vi "ini_Cylinder.vi"(8 "error IO":errorcluster) -> (0 "error out":errorcluster)   [LabVIEW 2017]
uses:
  Ctrls/AlarmIndex.ctl
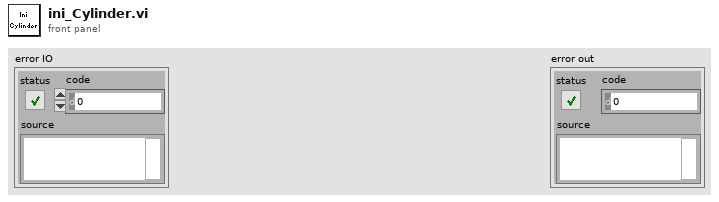
[diagram p1: front panel]
types:
  T1 = typedef "AlarmIndex.ctl" = enum16{"E-Stop", "Safety light grid", "UUT Sealing Cylinder HomePoint", "UUT Sealing Cylinder WorkPoint", "Orifice fixed Cylinder L HomePoint", "Orifice fixed Cylinder L WorkPoint", "Orifice fixed Cylinder R HomePoint", "Orifice fixed Cylinder R WorkPoint", "UUT Cylinder HomePoint", "UUT Cylinder WorkPoint", "Carrier fixed Cylinder L HomePoint", "Carrier fixed Cylinder L WorkPoint", "Carrier fixed Cylinder R HomePoint", "Carrier fixed Cylinder R WorkPoint", "Probe Cylinder HomePoint", "Probe Cylinder WorkPoint", "Motor Error", "Test Error"}
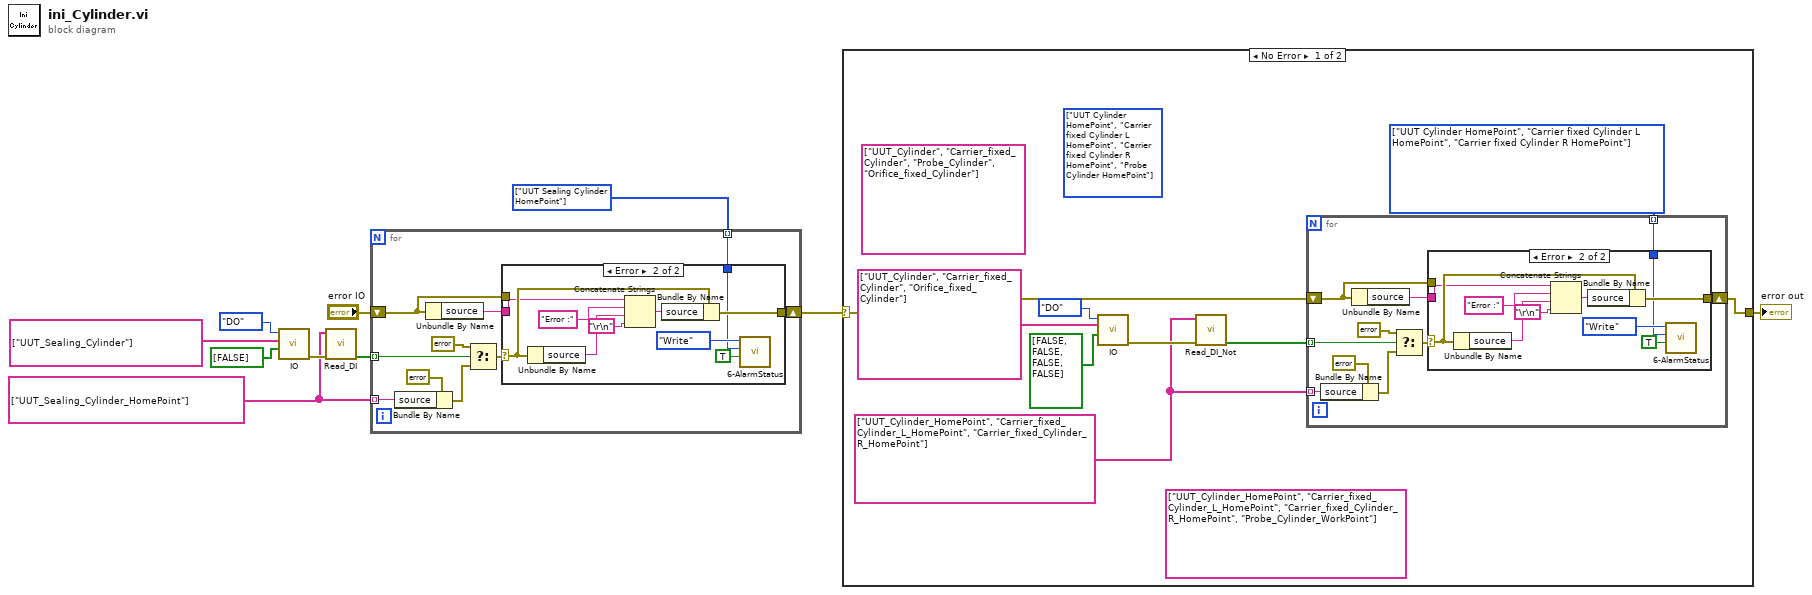
[diagram p0: block diagram]
diagram:
  w4 = T1[] [enum."UUT Sealing Cylinder HomePoint"] items=["E-Stop", "Safety light grid", "UUT Sealing Cylinder HomePoint", "UUT Sealing Cylinder WorkPoint", "Orifice fixed Cylinder L HomePoint", "Orifice fixed Cylinder L WorkPoint", "Orifice fixed Cylinder R HomePoint", "Orifice fixed Cylinder R WorkPoint", "UUT Cylinder HomePoint", "UUT Cylinder WorkPoint", "Carrier fixed Cylinder L HomePoint", "Carrier fixed Cylinder L WorkPoint", "Carrier fixed Cylinder R HomePoint", "Carrier fixed Cylinder R WorkPoint", "Probe Cylinder HomePoint", "Probe Cylinder WorkPoint", "Motor Error", "Test Error"]
  w5 = string[] ["UUT_Sealing_Cylinder_HomePoint"] ("IO Name")
  n1 = call "IO.vi"("DO DATA"=bool[] [FALSE] ("Writel_IO"), "IO Name"=string[] ["UUT_Sealing_Cylinder"], "IO?"=enum16{"DI", "DO"}."DO") -> ("error out"=w8:errorcluster)  [unwired: 7 in, 1 out]
  n2 = call "Read_DI.vi"("error in (no error)"=w8, "Name"=w5) -> ("DI"=w6:bool[])  [unwired: 8 in, 1 out]
  n3 = for {
    shift-right: [w16] -> w3
    shift-left: "error IO" -> [w12]
    tunnel: w6 -> [w18] mode=indexing
    tunnel: w5 -> [w15] mode=indexing
    tunnel: w4 -> [w11] mode=indexing
    n4 = Bundle By Name(cluster=errorcluster {"status"=TRUE, "code"=0, "source"=""} ("error out"), "source"=w15) -> (w17:errorcluster)
    n5 = Unbundle By Name(w12) -> ("source"=w13:string)
    n6 = Select(t=errorcluster {"status"=FALSE, "code"=0, "source"=""}, s=w18, f=w17) -> (s? t:f=w19:errorcluster)
    n7 = case shown="Error" w19 {
      selector: w19 -> [_ w27]
      tunnel: [w21 w31] -> w16
      tunnel: w13 -> [_ w25]
      tunnel: w12 -> [w21 _]
      tunnel: w11 -> [_ w23]
      frame No Error {
      }
      frame Error {
        n8 = Unbundle By Name(w27) -> ("source"=w29:string)
        n9 = Concatenate Strings(w25, "Error :" ("字符串"), w29, "\r\n") -> (w28:string)
        n10 = Bundle By Name(cluster=w27, "source"=w28) -> (w31:errorcluster)
        n11 = call "6-AlarmStatus.vi"("AlarmValue"=TRUE, "AlarmIndex"=w23, "Step"=enum16{"Initial", "Write", "Read"}."Write") -> ()  [unwired: 7 in, 2 out]
      }
    }
  }
  n12 = case shown="No Error" w3 {
    selector: w3 -> [w35 w62]
    tunnel: [w36 w62] -> w1
    frame No Error {
      (unwired) string[] ["UUT_Cylinder", "Carrier_fixed_Cylinder", "Probe_Cylinder", "Orifice_fixed_Cylinder"] ("IO Name")
      (unwired) T1[] [enum."UUT Cylinder HomePoint", enum."Carrier fixed Cylinder L HomePoint", enum."Carrier fixed Cylinder R HomePoint", enum."Probe Cylinder HomePoint"] items=["E-Stop", "Safety light grid", "UUT Sealing Cylinder HomePoint", "UUT Sealing Cylinder WorkPoint", "Orifice fixed Cylinder L HomePoint", "Orifice fixed Cylinder L WorkPoint", "Orifice fixed Cylinder R HomePoint", "Orifice fixed Cylinder R WorkPoint", "UUT Cylinder HomePoint", "UUT Cylinder WorkPoint", "Carrier fixed Cylinder L HomePoint", "Carrier fixed Cylinder L WorkPoint", "Carrier fixed Cylinder R HomePoint", "Carrier fixed Cylinder R WorkPoint", "Probe Cylinder HomePoint", "Probe Cylinder WorkPoint", "Motor Error", "Test Error"]
      (unwired) string[] ["UUT_Cylinder_HomePoint", "Carrier_fixed_Cylinder_L_HomePoint", "Carrier_fixed_Cylinder_R_HomePoint", "Probe_Cylinder_WorkPoint"] ("IO Name")
      w40 = T1[] [enum."UUT Cylinder HomePoint", enum."Carrier fixed Cylinder L HomePoint", enum."Carrier fixed Cylinder R HomePoint"] items=["E-Stop", "Safety light grid", "UUT Sealing Cylinder HomePoint", "UUT Sealing Cylinder WorkPoint", "Orifice fixed Cylinder L HomePoint", "Orifice fixed Cylinder L WorkPoint", "Orifice fixed Cylinder R HomePoint", "Orifice fixed Cylinder R WorkPoint", "UUT Cylinder HomePoint", "UUT Cylinder WorkPoint", "Carrier fixed Cylinder L HomePoint", "Carrier fixed Cylinder L WorkPoint", "Carrier fixed Cylinder R HomePoint", "Carrier fixed Cylinder R WorkPoint", "Probe Cylinder HomePoint", "Probe Cylinder WorkPoint", "Motor Error", "Test Error"]
      w33 = string[] ["UUT_Cylinder_HomePoint", "Carrier_fixed_Cylinder_L_HomePoint", "Carrier_fixed_Cylinder_R_HomePoint"] ("IO Name")
      n13 = call "IO.vi"("DO DATA"=bool[] [FALSE, FALSE, FALSE, FALSE] ("Writel_IO"), "IO Name"=string[] ["UUT_Cylinder", "Carrier_fixed_Cylinder", "Orifice_fixed_Cylinder"], "IO?"=enum16{"DI", "DO"}."DO") -> ("error out"=w34:errorcluster)  [unwired: 7 in, 1 out]
      n14 = call "Read_DI_Not.vi"("error in (no error)"=w34, "Name"=w33) -> ("DI"=w32:bool[])  [unwired: 8 in, 1 out]
      n15 = for {
        shift-right: [w46] -> w36
        shift-left: w35 -> [w42]
        tunnel: w32 -> [w48] mode=indexing
        tunnel: w33 -> [w45] mode=indexing
        tunnel: w40 -> [w41] mode=indexing
        n16 = Bundle By Name(cluster=errorcluster {"status"=TRUE, "code"=0, "source"=""} ("error out"), "source"=w45) -> (w47:errorcluster)
        n17 = Unbundle By Name(w42) -> ("source"=w43:string)
        n18 = Select(t=errorcluster {"status"=FALSE, "code"=0, "source"=""}, s=w48, f=w47) -> (s? t:f=w49:errorcluster)
        n19 = case shown="Error" w49 {
          selector: w49 -> [_ w57]
          tunnel: [w51 w61] -> w46
          tunnel: w43 -> [_ w55]
          tunnel: w42 -> [w51 _]
          tunnel: w41 -> [_ w53]
          frame No Error {
          }
          frame Error {
            n20 = Unbundle By Name(w57) -> ("source"=w59:string)
            n21 = Concatenate Strings(w55, "Error :" ("字符串"), w59, "\r\n") -> (w58:string)
            n22 = Bundle By Name(cluster=w57, "source"=w58) -> (w61:errorcluster)
            n23 = call "6-AlarmStatus.vi"("AlarmValue"=TRUE, "AlarmIndex"=w53, "Step"=enum16{"Initial", "Write", "Read"}."Write") -> ()  [unwired: 7 in, 2 out]
          }
        }
      }
    }
    frame Error {
    }
  }
  "error out" <- w1
